vi "Render Sidebar.vi"(8 "error in (no error)":errorcluster, 11 "Main Controller Actor in":refnum<class "Main Controller Actor.lvclass">) -> (0 "error out":errorcluster)   [LabVIEW 2021, in "Main Controller Actor.lvclass"]
uses:
  Main Controller Actor.lvclass
  Main Controller Actor.lvclass/Main Controller Actor.ctl
  LabSDL2/Source/Libraries/LibSDL2 Wrapper/Controls/Rectangle.ctl
  LabSDL2/Source/Libraries/LibSDL2 Wrapper/LibSDL2.lvlib
  Renderer/Renderer.lvclass
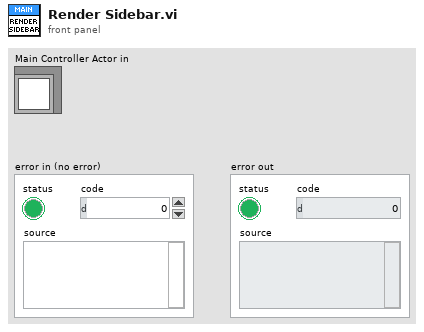
[diagram p1: front panel]
types:
  T1 = typedef "LibSDL2.lvlib/Rectangle.ctl" = cluster{"x":i32, "y":i32, "Width":i32, "Height":i32}
  T2 = typedef "Constants.ctl" = cluster{"Colours":cluster{"OK":u32, "Warning":u32, "Error":u32, "Red":u32, "Green":u32, "Blue":u32, "Yellow":u32}, "System":cluster{"Target Frames Second":dbl, "World Size":T3, "Window Size":T3, "Battle Area Size":T3, "Sidebar Scaling":sgl, "Sidebar Width":i32, "SC2 Frame Rate [Seconds/Frame]":sgl}, "Game":cluster{"Maximum Asteroids":i32, "Max Energy":i32, "Max Crew":i32, "Maximum Stars":i32}}
  T3 = typedef "SDL2 Utility.lvlib/Point (I32).ctl" = cluster{"x":i32, "y":i32}
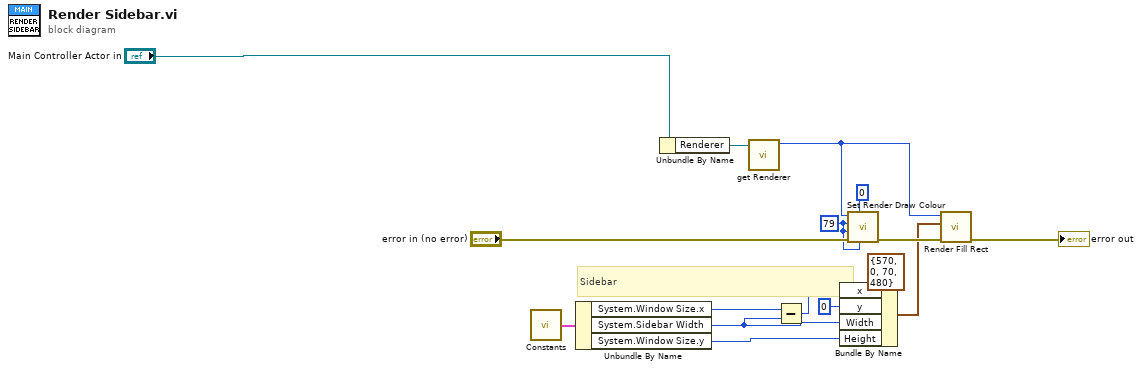
[diagram p0: block diagram]
diagram:
  w2 = u8 79 ("R")
  # "Sidebar"
  n1 = call "Constants.vi"() -> ("Constants"=w4:T2)
  n2 = Unbundle By Name(w4) -> ("System.Window Size.x"=w6:i32, "System.Sidebar Width"=w13:i32, "System.Window Size.y"=w7:i32)
  n3 = Unbundle By Name("Main Controller Actor in") -> ("Renderer"=w16:refnum<class "Renderer.lvclass">)
  n4 = call-dynamic "get Renderer.vi"("Renderer in"=w16) -> ("Renderer"=w14:u32)  [unwired: 10 in]
  n5 = Subtract(x=w6, y=w13) -> (x-y=w8:i32)
  n6 = Bundle By Name(cluster=T1 {"x"=570, "y"=0, "Width"=70, "Height"=480} ("Sidebar Colouring"), "x"=w8, "y"=0, "Width"=w13, "Height"=w7) -> (w9:T1)
  n7 = call "Set Render Draw Colour.vi"("B"=w2, "A"=u8 0, "error in (no error)"="error in (no error)", "G"=w2, "R"=w2, "Renderer Pointer"=w14) -> ("error out"=w10:errorcluster)  [unwired: 4 in, 1 out]
  n8 = call "Render Fill Rect.vi"("error in"=w10, "Rectangle"=w9, "Renderer Pointer"=w14) -> ("error out"=→"error out":errorcluster)  [unwired: 7 in, 1 out]
